vi "Scale_Motor.vi"(11 "Input":dbl) -> (3 "Output":dbl)   [LabVIEW 2013]
panel:
  in  "Scale":dbl
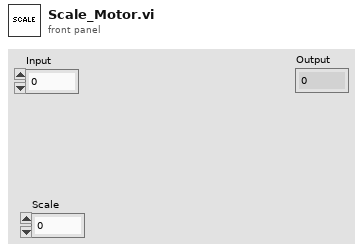
[diagram p1: front panel]
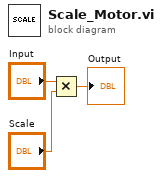
[diagram p0: block diagram]
diagram:
  n1 = Multiply(x="Input", y="Scale") -> (x*y=→"Output":dbl)
